vi "interface1.vi"() -> ()   [LabVIEW 2009]
panel:
  in  "stop":bool
  in  "get value":bool
  out "numeric":dbl
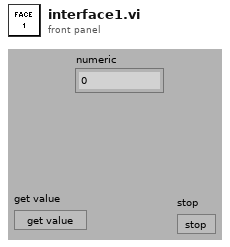
[diagram p1: front panel]
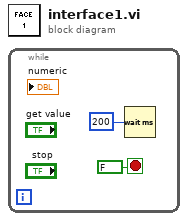
[diagram p0: block diagram]
diagram:
  n1 = while {
    stop <- FALSE stop-if-true
    n2 = Wait (ms)(milliseconds to wait=u32 200) -> ()  [unwired: 1 out]
  }
